vi "gyro_data_auto_modify.vi"() -> ()   [LabVIEW 2014]
uses:
  <vilib>/Platform/TimedLoop/XDataNode/timing_clust.ctl
  <vilib>/Platform/TimedLoop/XDataNode/nitl_modes.ctl
  <vilib>/Platform/TimedLoop/XDataNode/wakeup.ctl
  <vilib>/myRIO/Common/Instrument Driver Framework/myRIO v1.0/Encoder/typedefs/Encoder Signal Mode.ctl
  <vilib>/myRIO/Instrument Drivers/Onboard IO/Encoder/typedefs/Encoder Reference.ctl
  <vilib>/myRIO/Common/Instrument Driver Framework/Utilities/typedefs/myRIO Generic Hardware Reference.ctl
  <vilib>/myRIO/Common/Instrument Driver Framework/Utilities/typedefs/Hardware Version Enum.ctl
  <vilib>/myRIO/Common/Instrument Driver Framework/Utilities/typedefs/myRIO v1.0 Reference.ctl
  <vilib>/myRIO/Common/Instrument Driver Framework/Utilities/typedefs/Generic FPGA Reference.ctl
  <vilib>/myRIO/Common/Instrument Driver Framework/myRIO v1.0/Encoder/typedefs/Encoder Channels Enum.ctl
  <vilib>/myRIO/Common/Instrument Driver Framework/myRIO v1.0/Encoder/typedefs/Encoder Configuration v1.0.ctl
  <vilib>/userdefined/High Color/nirio_resource_hc.ctl
  <vilib>/Analysis/3filter.llb/Filter Passband Type.ctl
  <vilib>/myRIO/Common/Instrument Driver Framework/Utilities/vis/Is FPGA Ref Available.vi
  <vilib>/myRIO/Common/Instrument Driver Framework/myRIO v1.0/Encoder/vis/myRIO v1.1 Open Encoder.vi
  <vilib>/myRIO/Instrument Drivers/Onboard IO/Encoder/vis/Read.vi
  <vilib>/myRIO/Instrument Drivers/Onboard IO/PWM/vis/Set Duty Cycle and Frequency.vi
  <vilib>/myRIO/Instrument Drivers/Onboard IO/DIO/vis/Write.vi
  <vilib>/myRIO/Common/Instrument Driver Framework/Utilities/vis/Validate Channels.vi
  <vilib>/myRIO/Common/Instrument Driver Framework/myRIO v1.0/Encoder/vis/myRIO v1.0 Reserve Encoder.vi
  <vilib>/myRIO/Instrument Drivers/Onboard IO/AI/vis/Read.vi
  <vilib>/myRIO/Common/Instrument Driver Framework/myRIO v1.0/Encoder/vis/myRIO v1.0 Build MUX Configuration Encoder.vi
  <vilib>/myRIO/Common/Instrument Driver Framework/myRIO v1.0/Resource Manager/vis/myRIO v1.0 Reserve Channel List.vi
  <vilib>/myRIO/Common/Instrument Driver Framework/myRIO v1.0/Resource Manager/vis/myRIO v1.0 Create Configuration List.vi
  <vilib>/myRIO/Common/Instrument Driver Framework/myRIO v1.0/Resource Manager/vis/myRIO v1.0 Reserve Channel.vi
  <vilib>/myRIO/Common/Instrument Driver Framework/myRIO v1.0/Resource Manager/vis/myRIO v1.0 Unreserve Channel.vi
  <vilib>/myRIO/Common/Instrument Driver Framework/myRIO v1.0/Resource Manager/vis/myRIO v1.0 Build Mutex Name.vi
  <vilib>/myRIO/Instrument Drivers/Onboard IO/AI/vis/Smart Open.vi
  <vilib>/Utility/error.llb/Error Cluster From Error Code.vi
  <vilib>/myRIO/Common/Instrument Driver Framework/myRIO v1.0/AI/vis/myRIO v1.0 Read AI.vi
  <vilib>/myRIO/Instrument Drivers/Onboard IO/PWM/vis/Smart Open.vi
  <vilib>/myRIO/Common/Instrument Driver Framework/myRIO v1.0/PWM/vis/myRIO v1.0 Write PWM.vi
  <vilib>/myRIO/Instrument Drivers/Onboard IO/DIO/vis/Smart Open.vi
  <vilib>/myRIO/Common/Instrument Driver Framework/myRIO v1.0/DIO/vis/myRIO v1.0 Write DIO.vi
  <vilib>/addons/control/pid/pid.llb/PID (DBL).vi
  <vilib>/Utility/VariantDataType/GetNumericInfo.vi
  <vilib>/myRIO/Common/Instrument Driver Framework/myRIO v1.0/myRIO v1.1 Open.vi
  <vilib>/myRIO/Common/Instrument Driver Framework/Utilities/vis/IO Manager.vi
  <vilib>/myRIO/Common/Instrument Driver Framework/Utilities/vis/Configuration Manager.vi
  <vilib>/myRIO/Common/Instrument Driver Framework/myRIO v1.0/Resource Manager/vis/myRIO v1.0 Configure IO.vi
  <vilib>/myRIO/Common/Instrument Driver Framework/myRIO v1.0/myRIO v1.0 Close.vi
  <vilib>/myRIO/Common/Instrument Driver Framework/myRIO v1.0/Encoder/vis/myRIO v1.0 Configure Encoder.vi
  <vilib>/myRIO/Common/Instrument Driver Framework/myRIO v1.0/Encoder/vis/myRIO v1.0 Read Encoder.vi
  <vilib>/myRIO/Instrument Drivers/Onboard IO/Encoder/vis/Smart Open.vi
  <vilib>/Analysis/3filter.llb/Butterworth Filter (DBL).vi
  <vilib>/platform/TimedLoop/XDataNode/XDataNode.xnode
  <vilib>/myRIO/Express VI/Onboard IO/Encoder/Encoder Express VI.xnode
  <vilib>/myRIO/Instrument Drivers/Onboard IO/Encoder/vis/myRIO Encoder Open.xnode
  <vilib>/Platform/TimedLoop/XDataNode/XDNodeRunTimeDep.lvlib
  <vilib>/ptbypt/NI_PtbyPt.lvlib
  <vilib>/Analysis/NI_AALBase.lvlib
  <vilib>/myRIO/Instrument Drivers/Onboard IO/Encoder/Encoder.lvlib
  <vilib>/addons/control/pid/NI_PID_pid.lvlib
panel:
  in  "关闭程序":bool
  in  "A_Duty":dbl(slide) scale=-1.0..1.0
  in  "B_Duty":dbl(slide) scale=-1.0..1.0
  in  "电机开关":bool
  out "position_A":i32
  in  "Reset_A":bool
  out "Average_A":dbl(graph)
  out "position_B":i32
  in  "Reset_B":bool
  out "velocity_B":dbl(graph)
  out "Average_B":dbl(graph)
  out "t-time":dbl
  out "gyro_bias":dbl
  out "Angluar Rate 3":dbl
  out "Angle_org 2":dbl(graph)
  in  "initialize_org 2":bool
  out "Angluar Rate 2":dbl(graph)
  out "time":dbl
  out "Angluar Rate":dbl
  out "文件路径":path
  out "Angle_org":dbl(graph)
  in  "initialize_org":bool
  in  "initialize_Butterworth":bool
  out "Angle_Butterworth":dbl(graph)
  out "Angluar Rate_Butterworth":dbl(graph)
  out "Angle_average":dbl(graph)
  in  "initialize_average":bool
  out "Angluar Rate_average":dbl(graph)
  out "Angluar Rate":dbl(graph)
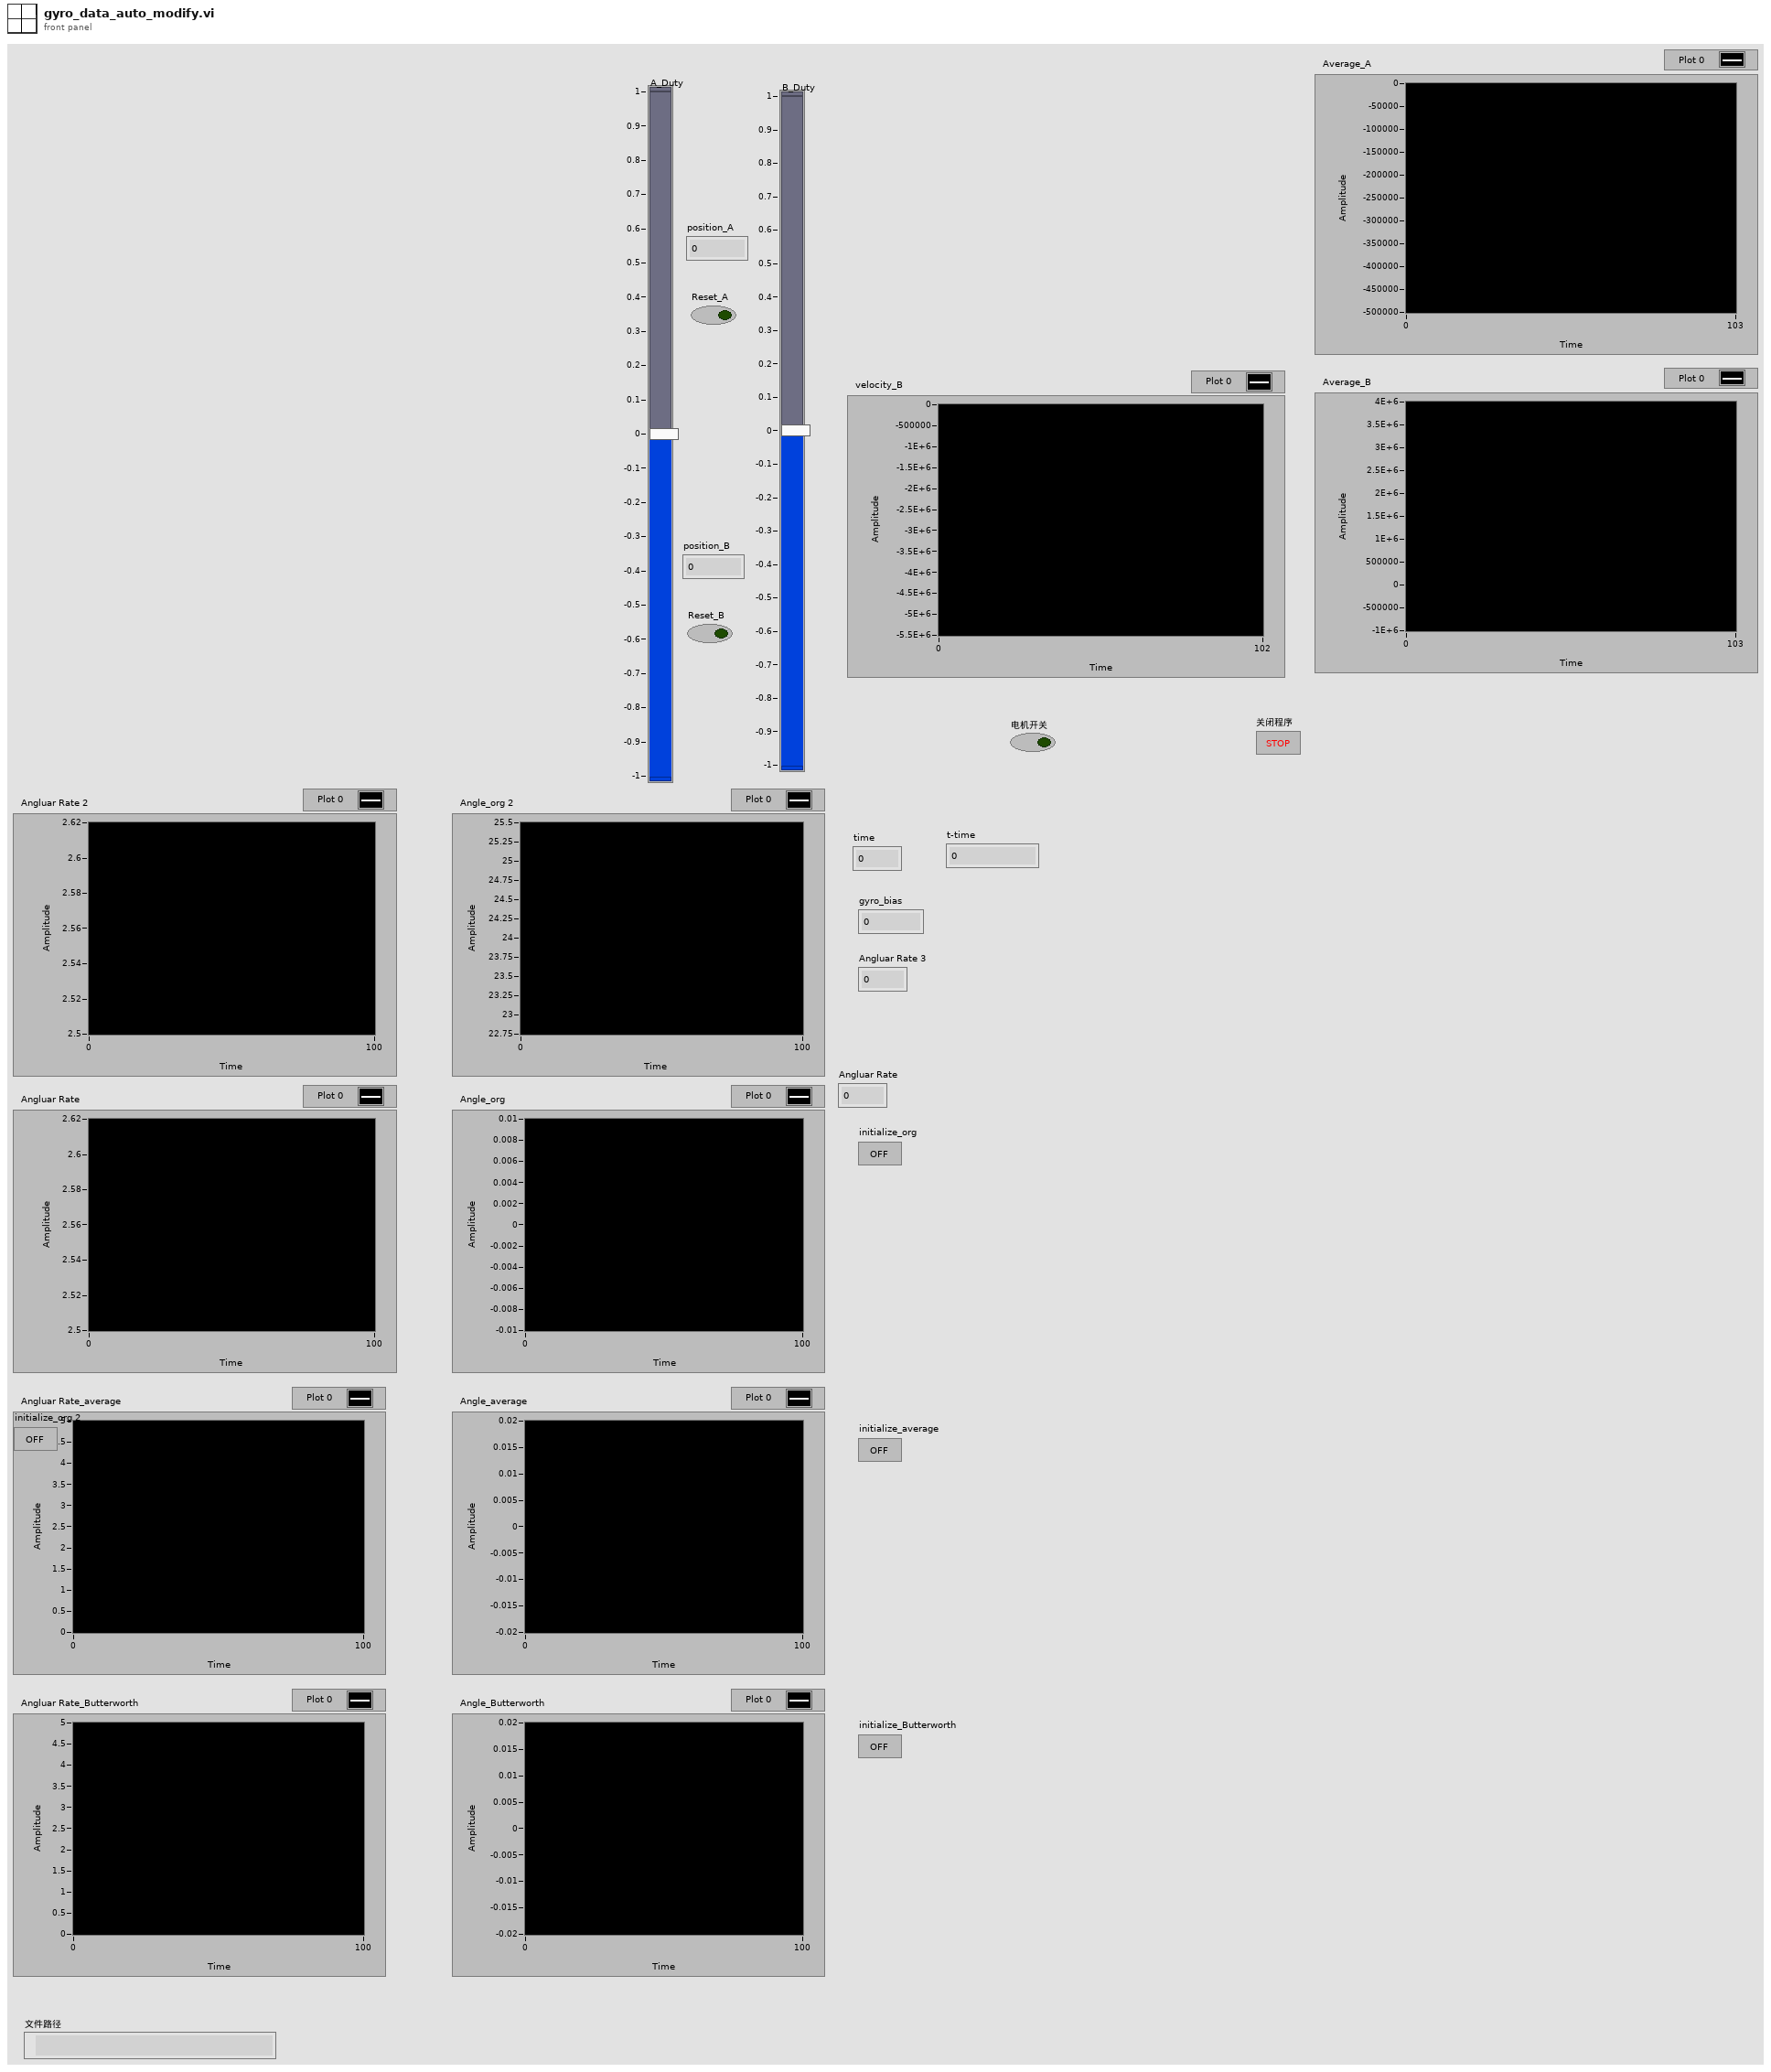
[diagram p1: front panel]
types:
  T1 = enum16{"open", "replace", "create", "open or create", "replace or create", "replace or create with confirmation"}
  T2 = typedef "XDNodeRunTimeDep.lvlib/timing_clust.ctl" = cluster{"Expected End [f-1]":u64, "Actual End [f-1]":u64, "Finished Late? [f-1]":bool, "Expected End [i-1]":u64, "Actual End [i-1]":u64, "Finished Late? [i-1]":bool, "Expected Start [i]":u64, "Actual Start [i]":u64, "Expected Start [f]":u64, "Actual Start [f]":u64, "Source Name":string, "Structure Name":string, "Period":i64, "Deadline":i64, "Offset":i64, "Start":i64, "Priority":i32, "Timeout":i32, "Mode":T3, "Wakeup Reason":T4, "Error":errorcluster, "Source Type":string, "Secondary Source Type":string, "Global End Time":u64, "Global Start Time":u64, "Frame Duration":u64, "Iteration Duration":u64, "Assigned CPU":i32, "I/O Scan Engine Mode":u32}
  T3 = typedef "XDNodeRunTimeDep.lvlib/nitl_modes.ctl" = enum32{"No Change", "Process missed periods, maintain original phase", "Discard missed periods, maintain original phase", "Process missed periods, ignore original phase", "Discard missed periods, ignore original phase"}
  T4 = typedef "XDNodeRunTimeDep.lvlib/wakeup.ctl" = enum32{"Normal", "Aborted", "Asynchronous wakeup", "Timing source error", "Timed loop error", "Timeout"}
  T5 = typedef "NI_AALBase.lvlib/Filter Passband Type.ctl" = enum32{"Lowpass", "Highpass", "Bandpass", "Bandstop"}
  T6 = typedef "Encoder.lvlib/Encoder Reference.ctl" = cluster{"myRIO Reference":T7, "Encoder Channels Enum":T11}
  T7 = typedef "myRIO Generic Hardware Reference.ctl" = cluster{"myRIO Model":T8, "myRIO Hardware Reference":T9}
  T8 = typedef "Hardware Version Enum.ctl" = enum16{"Unknown", "myRIO-1900", "myRIO-1950"}
  T9 = typedef "myRIO v1.0 Reference.ctl" = cluster{"Generic FPGA Reference":T10, "Allow multiple opens":bool}
  T10 = typedef "Generic FPGA Reference.ctl" = refnum<k20>
  T11 = typedef "Encoder Channels Enum.ctl" = enum16{"Not Connected", "C/ENC0", "C/ENC1", "A/ENC", "B/ENC"}
  T12 = typedef "Encoder Signal Mode.ctl" = enum16{"Quadrature phase signal", "Step and direction signal"}
  T13 = typedef "nirio_resource_hc.ctl" = tag
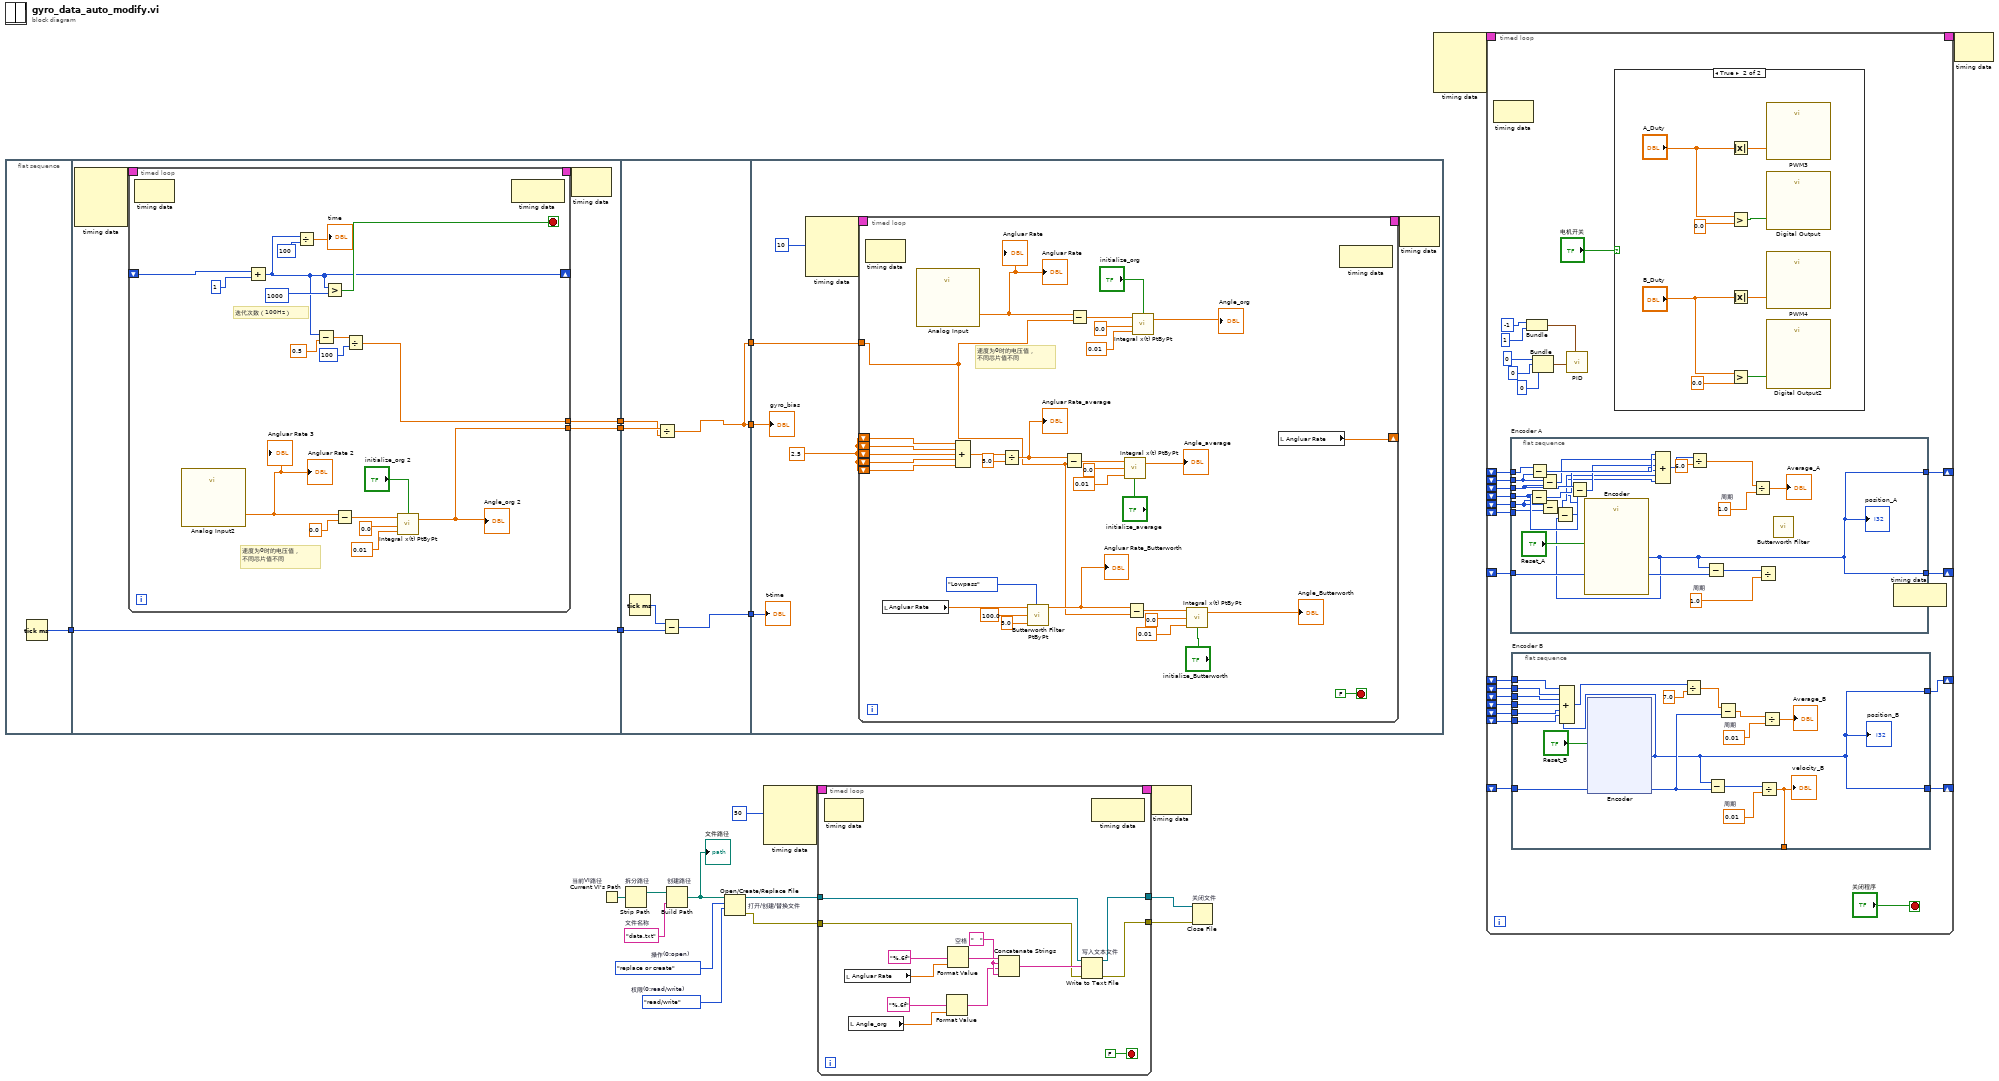
[diagram p0: block diagram]
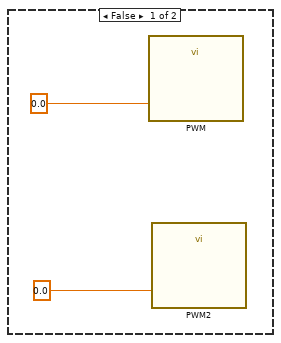
[diagram p2: hidden frame]
diagram:
  w20 = "data.txt"  # 文件名称
  w21 = enum16{"read/write", "read-only", "write-only"}."read/write"  # 权限(0:read/write)
  w22 = T1."replace or create"  # 操作(0:open)
  n1 = flat-sequence {
    tunnel: [w23] -> w5
    tunnel: [w26] -> w9
    tunnel: [w25] -> w6
    tunnel: w5 -> [w25]
    tunnel: [w24] -> w3
    tunnel: w9 -> [w56]
    tunnel: [w52] -> w8
    tunnel: [w53] -> w7
    tunnel: w6 -> [w54]
    tunnel: [w52] -> w4
    tunnel: w3 -> [w51]
    tunnel: w8 -> [w59]
    tunnel: w7 -> [w58]
    tunnel: w4 -> [w57]
    frame #0 {
      n2 = Tick Count (ms)() -> (millisecond timer value=w23:u32)
    }
    frame #1 {
      n3 = node-c288() -> (w28:T2)  [unwired: 4 in]
      n4 = timed-loop {
        timing: w28 -> [_]
        timing-out: [_] -> w27
        shift-right: [w33] -> _
        shift-left: _ -> [w45]
        tunnel: [w36] -> w26
        tunnel: [w29] -> w24
        stop <- w43 stop-if-true
        # "迭代次数（100Hz）"
        # "速度为0时的电压值，\n不同芯片值不同"
        n5 = node-c288() -> ()  [unwired: 1 in, 1 out]
        n6 = call "Analog Input2"() -> ("B/AI0 (Pin 3)"=w38:dbl)  [unwired: 26 in, 1 out]
        "Angluar Rate 2" <- w38
        "Angluar Rate 3" <- w38
        n7 = Add(x=w45, y=1) -> (x+y=w33:i32)
        n8 = Divide(x=w33, y=100) -> (x/y=→"time":dbl)
        n9 = Subtract(x=w33, y=0.5) -> (x-y=w31:dbl)
        n10 = Greater?(x=w33, y=1000 ("等待时间")) -> (0:w43:bool)
        n11 = Subtract(x=w38, y=0.0) -> (x-y=w42:dbl)
        n12 = Divide(x=w31, y=100) -> (x/y=w29:dbl)
        n13 = call <vilib>:"Integral x(t) PtByPt.vi"("initialize"="initialize_org 2", "dt"=0.01, "initial condition"=0.0, "x"=w42) -> ("integral x(t)"=w36:dbl)  [unwired: 1 out]
        "Angle_org 2" <- w36
        n14 = node-c288() -> ()  [unwired: 1 in, 1 out]
      }
      n15 = node-c288(w27) -> ()  [unwired: 1 out]
    }
    frame #2 {
      n16 = Tick Count (ms)() -> (millisecond timer value=w55:u32)
      n17 = Divide(x=w56, y=w51) -> (x/y=w52:dbl)
      n18 = Subtract(x=w55, y=w54) -> (x-y=w53:u32)
    }
    frame #3 {
      w61 = 2.5
      n19 = node-c288(i64 10 ("Period")) -> (w63:T2)  [unwired: 3 in]
      n20 = timed-loop {
        shift-right: [w69] -> _
        shift-left: w61 -> [w95]
        shift-left: w61 -> [w94]
        shift-left: w61 -> [w93]
        shift-left: w61 -> [w92]
        shift-left: w61 -> [w91]
        timing: w63 -> [_]
        timing-out: [_] -> w62
        tunnel: w59 -> [w64]
        stop <- FALSE stop-if-true
        # "速度为0时的电压值，\n不同芯片值不同"
        n21 = node-c288() -> ()  [unwired: 1 in, 1 out]
        n22 = local read "Angluar Rate"() -> (w78:dbl)
        n23 = call "Analog Input"() -> ("B/AI0 (Pin 3)"=w68:dbl)  [unwired: 26 in, 1 out]
        "Angluar Rate" <- w68
        "Angluar Rate" <- w68
        n24 = Compound Arithmetic op=ADD(w95, w94, w93, w92, w91) -> (w90:dbl)
        n25 = Divide(x=w90, y=5.0) -> (x/y=w79:dbl)
        "Angluar Rate_average" <- w79
        n26 = call <vilib>:"Butterworth Filter PtByPt.vi"("filter type"=Filter_Passband_Type."Lowpass", "low cutoff freq: fl"=5.0, "sampling freq: fs"=100.0, "x"=w78) -> ("Filtered x"=w73:dbl)  [unwired: 5 in, 1 out]
        "Angluar Rate_Butterworth" <- w73
        n27 = Subtract(x=w79, y=w64) -> (x-y=w87:dbl)
        n28 = Subtract(x=w68, y=w64) -> (x-y=w72:dbl)
        n29 = call <vilib>:"Integral x(t) PtByPt.vi"("initialize"="initialize_average", "dt"=0.01, "initial condition"=0.0, "x"=w87) -> ("integral x(t)"=→"Angle_average":dbl)  [unwired: 1 out]
        n30 = Subtract(x=w73, y=w64) -> (x-y=w74:dbl)
        n31 = call <vilib>:"Integral x(t) PtByPt.vi"("initialize"="initialize_org", "dt"=0.01, "initial condition"=0.0, "x"=w72) -> ("integral x(t)"=→"Angle_org":dbl)  [unwired: 1 out]
        n32 = call <vilib>:"Integral x(t) PtByPt.vi"("initialize"="initialize_Butterworth", "dt"=0.01, "initial condition"=0.0, "x"=w74) -> ("integral x(t)"=→"Angle_Butterworth":dbl)  [unwired: 1 out]
        n33 = local read "Angluar Rate"() -> (w69:dbl)
        n34 = node-c288() -> ()  [unwired: 1 in, 1 out]
      }
      n35 = node-c288(w62) -> ()  [unwired: 1 out]
      "t-time" <- w58
      "gyro_bias" <- w57
    }
  }
  n36 = Current VI's Path "当前VI路径"() -> (path=w19:path)
  n37 = Strip Path "拆分路径"(path=w19) -> (stripped path=w18:path)  [unwired: 1 out]
  n38 = Build Path "创建路径"(base path=w18, name or relative path=w20) -> (appended path=w17:path)
  "文件路径" <- w17
  n39 = Open/Create/Replace File "打开/创建/替换文件"(file path (use dialog)=w17, operation (0:open)=w22, access (0:read/write)=w21) -> (refnum out=w12:refnum<file>, error out=w11:errorcluster)  [unwired: 1 in, 3 out]
  n40 = node-c288(50 ("Priority")) -> (w16:T2)  [unwired: 3 in]
  n41 = timed-loop {
    timing: w16 -> [_]
    timing-out: [_] -> w15
    tunnel: w12 -> [w111]
    tunnel: w11 -> [w110]
    tunnel: [w108] -> w14
    tunnel: [w107] -> w13
    stop <- FALSE stop-if-true
    w103 = "   "  # 空格
    n42 = node-c288() -> ()  [unwired: 1 in, 1 out]
    n43 = local read "Angluar Rate"() -> (w106:dbl)
    n44 = local read "Angle_org"() -> (w105:dbl)
    n45 = Format Value(format string="%.6f", value (0)=w105) -> (output string=w102:string)  [unwired: 1 in]
    n46 = Format Value(format string="%.6f", value (0)=w106) -> (output string=w113:string)  [unwired: 1 in]
    n47 = Concatenate Strings(w113, w103, w102, w103) -> (w112:string)
    n48 = Write to Text File "写入文本文件"(file (use dialog)=w111, text=w112, error in=w110) -> (refnum out=w108:refnum<file>, error out=w107:errorcluster)  [unwired: 2 out]
    n49 = node-c288() -> ()  [unwired: 1 in, 1 out]
  }
  n50 = node-c288(w15) -> ()  [unwired: 1 out]
  n51 = Close File "关闭文件"(refnum=w14, error in=w13) -> ()  [unwired: 2 out]
  n52 = node-c288() -> (w2:T2)  [unwired: 4 in]
  n53 = timed-loop {
    timing: w2 -> [_]
    timing-out: [_] -> w1
    shift-right: [w141] -> _
    shift-left: _ -> [w140]
    shift-right: [w138] -> _
    shift-left: _ -> [w139]
    shift-right: [w136] -> _
    shift-left: _ -> [w137]
    shift-left: _ -> [w133]
    shift-left: _ -> [w135]
    shift-left: _ -> [w134]
    shift-left: _ -> [w132]
    shift-left: _ -> [w131]
    shift-right: [w129] -> _
    shift-left: _ -> [w124]
    shift-left: _ -> [w126]
    shift-left: _ -> [w128]
    shift-left: _ -> [w125]
    shift-left: _ -> [w127]
    shift-left: _ -> [w130]
    stop <- "关闭程序" stop-if-true
    n54 = node-c288() -> ()  [unwired: 1 in, 1 out]
    n55 = flat-sequence "Encoder A" {
      tunnel: [w215] -> w141
      tunnel: w140 -> [w223]
      tunnel: w130 -> [w219]
      tunnel: [w215] -> w129
      tunnel: w128 -> [w218]
      tunnel: w127 -> [w217]
      tunnel: w126 -> [w216]
      tunnel: w125 -> [w220]
      tunnel: w124 -> [w221]
      frame #0 {
        w226 = 1.0  # 周期
        w227 = 1.0  # 周期
        n56 = Subtract(x=w218, y=w217) -> (x-y=w211:i32)
        n57 = Subtract(x=w221, y=w220) -> (x-y=w214:i32)
        n58 = Subtract(x=w220, y=w219) -> (x-y=w213:i32)
        n59 = Subtract(x=w217, y=w216) -> (x-y=w210:i32)
        n60 = Subtract(x=w219, y=w218) -> (x-y=w212:i32)
        n61 = call "Encoder"("Reset Counter"="Reset_A") -> ("Counter Value"=w215:i32)  [unwired: 23 in, 3 out]
        "position_A" <- w215
        n62 = Subtract(x=w216, y=w215) -> (x-y=w209:i32)
        n63 = Compound Arithmetic op=ADD(w214, w213, w212, w211, w210, w209) -> (w222:i32)
        n64 = Divide(x=w222, y=6.0) -> (x/y=w208:dbl)
        n65 = Subtract(x=w215, y=w223) -> (x-y=w228:i32)
        n66 = Divide(x=w208, y=w226) -> (x/y=→"Average_A":dbl)
        n67 = Divide(x=w228, y=w227) -> ()  [unwired: 1 out]
        n68 = call-poly <vilib>:"Butterworth Filter.vi"() -> ()  [unwired: 8 in, 2 out]
      }
    }
    n69 = flat-sequence "Encoder B" {
      tunnel: [w144] -> w138
      tunnel: w139 -> [w151]
      tunnel: [w159] -> _
      tunnel: w137 -> [w158]
      tunnel: [w144] -> w136
      tunnel: w135 -> [w157]
      tunnel: w134 -> [w156]
      tunnel: w133 -> [w147]
      tunnel: w132 -> [w146]
      tunnel: w131 -> [w145]
      frame #0 {
        w149 = 0.01  # 周期
        w160 = 0.01  # 周期
        n70 = xnode "Encoder"("Reset Counter"="Reset_B") -> ("Counter Value"=w144:i32)  [unwired: 1 in, 3 out]
        "position_B" <- w144
        n71 = Compound Arithmetic op=ADD(w158, w157, w156, w147, w146, w145, w144) -> (w154:i32)
        n72 = Divide(x=w154, y=7.0) -> (x/y=w152:dbl)
        n73 = Subtract(x=w144, y=w151) -> (x-y=w161:i32)
        n74 = Subtract(x=w152, y=w151) -> (x-y=w150:dbl)
        n75 = Divide(x=w161, y=w160) -> (x/y=w159:dbl)
        "velocity_B" <- w159
        n76 = Divide(x=w150, y=w149) -> (x/y=→"Average_B":dbl)
      }
    }
    n77 = Bundle(-1, 1) -> (w119:cluster{i32, i32})  [unwired: 1 in]
    n78 = Bundle(0, 0, 0) -> (w120:cluster{i32, i32, i32})  [unwired: 1 in]
    n79 = call-poly <vilib>:"PID.vi"("output range"=w119, "PID gains"=w120) -> ()  [unwired: 8 in, 2 out]
    n80 = case shown="True" "电机开关" {
      frame False {
        n81 = call "PWM"("Duty Cycle (0-1)"=0.0) -> ()  [unwired: 26 in, 1 out]
        n82 = call "PWM2"("Duty Cycle (0-1)"=0.0) -> ()  [unwired: 26 in, 1 out]
      }
      frame True {
        n83 = Absolute Value(x="A_Duty") -> (abs(x)=w237:dbl)
        n84 = Greater?(x="A_Duty", y=0.0) -> (0:w238:bool)
        n85 = Absolute Value(x="B_Duty") -> (abs(x)=w233:dbl)
        n86 = Greater?(x="B_Duty", y=0.0) -> (0:w232:bool)
        n87 = call "PWM3"("Duty Cycle (0-1)"=w237) -> ()  [unwired: 26 in, 1 out]
        n88 = call "Digital Output"("A/DIO0 (Pin 11)"=w238) -> ()  [unwired: 26 in, 1 out]
        n89 = call "PWM4"("Duty Cycle (0-1)"=w233) -> ()  [unwired: 26 in, 1 out]
        n90 = call "Digital Output2"("B/DIO0 (Pin 11)"=w232) -> ()  [unwired: 26 in, 1 out]
      }
    }
    n91 = node-c288() -> ()  [unwired: 1 in, 1 out]
  }
  n92 = node-c288(w1) -> ()  [unwired: 1 out]
